vi "RT Driver VI.vi"(7 "Operation":T1, 11 "Device Reference in":T2 format="%.0x") -> (0 "Error Code":i32)   [LabVIEW 2021, in "FPGA Addon Engine.lvlib"]
uses:
  FPGA Addon Engine.lvlib
  <vilib>/NI VeriStand/Custom Device API/Custom Device Item Ref.ctl
  <vilib>/NI VeriStand/Custom Device API/Hardware Interface Driver VI Operation.ctl
  <vilib>/NI/NIVS Inline Async API/_VS Inline Async API/VS Inline Async API/Types/Error Handling Settings.ctl
  <vilib>/NI/NIVS Inline Async API/_VS Inline Async API/VS Inline Async API/VS Inline Async API.lvclass/VS Inline Async API.ctl
  <vilib>/NI/NIVS Inline Async API/_Data Access Engine/Data Access Engine/Data Access Engine.lvclass/Data Access Engine.ctl
  <vilib>/NI/NIVS Inline Async API/_Data Access Engine/Access Type Classes/Write/Write.lvclass/Write.ctl
  <vilib>/NI/NIVS Inline Async API/_Data Access Engine/Access Type Classes/ReadWrite/ReadWrite.lvclass/ReadWrite.ctl
  <vilib>/NI/NIVS Inline Async API/_Data Access Engine/Access Type Classes/Read/Read.lvclass/Read.ctl
  Addon Shared/SubVIs/FPGA Settings.vi
  SubVIs/Initialize Scalar Datatypes and Refs.vi
  <vilib>/NI/NIVS Inline Async API/_Data Access Engine/Data Access Engine/Methods/Data.Engine.Read Data from HW.vi
  <vilib>/NI/NIVS Inline Async API/_VS Inline Async API/Error Handling Process/SubVIs/Error.GetError.vi
  <vilib>/NI/NIVS Inline Async API/_Data Access Engine/Data Access Engine/Methods/Data.Engine.Write Data to HW.vi
  <vilib>/NI/NIVS Inline Async API/_Data Access Engine/Access Type Classes/ReadWrite/ReadWrite.EngineData.vi
  <vilib>/NI/NIVS Inline Async API/_Data Access Engine/Access Type Classes/Write/Write.EngineData.vi
  <vilib>/NI/NIVS Inline Async API/_Data Access Engine/Access Type Classes/Read/Read.EngineData.vi
  <vilib>/NI VeriStand/Custom Device API/NI VeriStand - Get Channel Value by Data Reference.vi
  <vilib>/NI VeriStand/Custom Device API/NI VeriStand - Set Channel Value by Data Reference.vi
  <vilib>/NI VeriStand/Custom Device API/NI VeriStand - Get Target Type.vi
  <vilib>/Utility/config.llb/Open Config Data.vi
  <vilib>/Utility/config.llb/Get Key Names.vi
  <vilib>/Utility/config.llb/Write Key.vi
  <vilib>/Utility/config.llb/Write Key (I32).vi
  <vilib>/Utility/config.llb/Close Config Data.vi
  <vilib>/NI VeriStand/Custom Device API/NI VeriStand - Get Item Property.vi
  <vilib>/NI VeriStand/Custom Device API/Get Item Property (Variant).vi
  <vilib>/NI VeriStand/Custom Device API/Get Item Property (Dependent File).vi
  <vilib>/NI VeriStand/Custom Device API/Get Item Property (Path).vi
  <vilib>/NI VeriStand/Custom Device API/Get Item Property (String).vi
  <vilib>/NI VeriStand/Custom Device API/Get Item Property (Boolean).vi
  <vilib>/NI VeriStand/Custom Device API/NI VeriStand - Set Item Property.vi
  <vilib>/NI VeriStand/Custom Device API/Set Item Property (Path).vi
  <vilib>/NI VeriStand/Custom Device API/Set Item Property (String).vi
  <vilib>/NI VeriStand/Custom Device API/Set Item Property (Boolean).vi
  APIs/FPGA Register IO/Utilities/Open FPGA Session.vi
  SubVIs/Initialize Input DMA Refs.vi
  SubVIs/Initialize Output DMA Refs.vi
  SubVIs/Initialize Scalar Datatype Classes.vi
  <vilib>/Utility/SystemLogging/Write to System Log.vi
  Processes/Input Registers Engine.vi
  Processes/Output Registers Engine.vi
  Processes/Output DMA Engine.vi
  Processes/Input DMA Engine.vi
  <vilib>/Utility/error.llb/Error Cluster From Error Code.vi
  <vilib>/RVI Host/nirviSupport.llb/nirviErrorClusterFromErrorCode.vi
  <vilib>/rvi/errors/niLvFpgaAdjustHostInterfaceError.vi
  <vilib>/NI VeriStand/Custom Device API/Global Data Refs.vi
  <vilib>/FPGAPlugInAG/Dynamic/niLvFpga_Close_Dynamic.vi
  <vilib>/NI VeriStand/Custom Device Waveform API/Multiple Waveforms Write (DBL)/Multiple Waveforms Write (DBL).lvclass
  <vilib>/NI VeriStand/Custom Device Waveform API/Single Waveform Read (DBL)/Single Waveform Read (DBL).lvclass
  <vilib>/NI/NIVS Inline Async API/_VS Inline Async API/VS Inline Async API/VS Inline Async API.lvclass
  <vilib>/rvi/interface/nirviMethod/nirviMethod.xnode
  <vilib>/rvi/interface/nirviCloseFPGA/nirviCloseFPGA.xnode
  <vilib>/NI VeriStand/Custom Device API/Custom Device API.lvlib
  <vilib>/rvi/interface/nirviMethod/StockFPGA_InlinedMethodWaitForSingleIRQ.vi
  <vilib>/FPGAPlugInAG/Dynamic/niLvFpga_WaitOnIrq_Dynamic.vi
  <vilib>/FPGAPlugInAG/Dynamic/niLvFpga_AcknowledgeIrq_Dynamic.vi
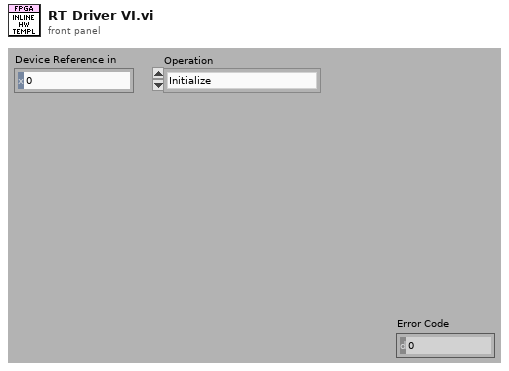
[diagram p1: front panel]
types:
  T1 = typedef "Custom Device API.lvlib/Hardware Interface Driver VI Operation.ctl" = enum16{"Initialize", "Start", "Read Data from HW", "Write Data to HW", "Close"}
  T2 = typedef "Custom Device API.lvlib/Custom Device Item Ref.ctl" = u64
  T3 = typedef "FPGA Addon Engine.lvlib/State Variables.ctl" = cluster{"FPGA Ref":refnum<k20>, "IncomingRegisters.Refs":T4[], "IncomingDMA.Refs":T7[], "OutgoingRegisters.Refs":T4[], "OutgoingDMA.Refs":T12[], "Compiled":T14}
  T4 = typedef "FPGA Addon Engine.lvlib/Register Settings.ctl" = cluster{"Name":string, "Data Type":T5, "session":u32, "Scalar Type":T6, "Index":i32, "Length":i32, "attributes":variant, "default value":variant}
  T5 = typedef "FPGA Addon Shared.lvlib/FPGA Addon Data Type.ctl" = enum8{"<Null>", "I8", "I16", "I32", "I64", "U8", "U16", "U32", "U64", "SGL", "Boolean", "Analog PWM In Settings", "Analog PWM In", "Digital PWM In Settings", "Digital PWM In", "Digital PWM Out", "Sine Out", "FXP", "FXP+/-24.5", "FXP+/-16.5", "FXP+/-32.8", "FXP+/-64.32", "FXP+/-16.7", "FXP+/-20.5", "FXP+/-27.5", "FXP+/-32.16", "FXP+16.3", "FXP+18.3", "Digital Static In", "Digital Static Out", "Digital Static In Settings", "Digital WSS Out", "Quad Encoder Settings", "Quad Encoder In", "Group"}
  T6 = typedef "FPGA Addon Shared.lvlib/Scalar Type.ctl" = enum16{"Standard", "Bitpacked"}
  T7 = typedef "FPGA Addon Engine.lvlib/DMA Input References.ctl" = cluster{"Addon Name":string, "Waveform Ref":refnum<class "Multiple Waveforms Write (DBL).lvclass">, "DMA Name":string, "DMA Settings":T8, "Refs":T11}
  T8 = typedef "FPGA Addon Shared.lvlib/DMA Settings.ctl" = cluster{"Number of Channels":u8, "Delacing Scheme":T9, "Update Rate":u32, "dt":dbl, "Mode":T10, "Number of Samples":u32, "DMA Host Buffer":u32}
  T9 = typedef "FPGA Addon Shared.lvlib/Delacing Scheme.ctl" = enum8{"Interleaved", "Bitpacked"}
  T10 = typedef "FPGA Addon Shared.lvlib/DMA Acquisition Mode.ctl" = enum8{"Continuous", "Triggered Finite"}
  T11 = typedef "FPGA Addon Engine.lvlib/DMA Input Refs.ctl" = cluster{"Data Type":T5, "DMA_SGL":refnum<k20>, "DMA_U64":refnum<k20>, "DMA_I64":refnum<k20>, "DMA_FXP+/-32.8":refnum<k20>, "DMA_FXP+/-64.32":refnum<k20>, "DMA_U32":refnum<k20>, "DMA_U16":refnum<k20>, "DMA_U8":refnum<k20>, "DMA_I32":refnum<k20>, "DMA_I16":refnum<k20>, "DMA_I8":refnum<k20>, "DMA_FXP+/-32.16":refnum<k20>}
  T12 = typedef "FPGA Addon Engine.lvlib/DMA Output References.ctl" = cluster{"Addon Name":string, "Waveforms":refnum<class "Single Waveform Read (DBL).lvclass">[], "DMA Name":string, "Refs":T13}
  T13 = typedef "FPGA Addon Engine.lvlib/DMA Output Refs.ctl" = cluster{"Data Type":T5, "DMA_SGL":refnum<k20>, "DMA_U64":refnum<k20>, "DMA_I64":refnum<k20>, "DMA_FXP+/-32.8":refnum<k20>, "DMA_FXP+/-64.32":refnum<k20>, "DMA_U32":refnum<k20>, "DMA_U16":refnum<k20>, "DMA_U8":refnum<k20>, "DMA_I32":refnum<k20>, "DMA_I16":refnum<k20>, "DMA_I8":refnum<k20>, "DMA_FXP+/-32.16":refnum<k20>}
  T14 = typedef "FPGA Addon Shared.lvlib/Compiled.Settings.ctl" = cluster{"Name":string, "IncomingRegisters.Settings":T15[], "IncomingRegisters.Refs":cluster{"Refs":T17[], "Values":dbl[]}, "OutgoingRegisters.Settings":T15[], "OutgoingRegisters.Refs":cluster{"Refs":T17[], "Values":dbl[]}, "Incoming.Size":i32, "Outgoing.Size":i32, "IncomingDMA.Settings":T19[], "OutgoingDMA.Settings":T19[], "FPGA.Settings":T21, "Target.Type":T22}
  T15 = typedef "FPGA Addon Shared.lvlib/Compiled.RegisterSettings.ctl" = cluster{"Scalar Type":T6, "Index":i32, "Length":i32, "Register":T16}
  T16 = typedef "FPGA Addon Shared.lvlib/Register Information.ctl" = cluster{"Name":string, "Data Type":T5, "Default Value":variant, "Attributes":variant}
  T17 = typedef "Custom Device API.lvlib/Block Data Reference.ctl" = cluster{"Data Reference":T18, "Offset":u64, "Length":u64}
  T18 = typedef "Custom Device API.lvlib/Data Reference.ctl" = i32
  T19 = typedef "FPGA Addon Shared.lvlib/Compiled.DMASettings.ctl" = cluster{"Name":string, "Data Type":T5, "DMA.Settings":T8, "DMA.VSRefs":T20[]}
  T20 = typedef "Custom Device API.lvlib/Waveform Data Reference.ctl" = i32
  T21 = typedef "FPGA Addon Shared.lvlib/FPGA Settings.ctl" = cluster{"Bitfile path":path, "RIO Device Address":string, "Group":bool}
  T22 = typedef "Custom Device API.lvlib/Custom Device Target Type.ctl" = enum16{"PharLap", "VxWorks", "Windows", "Linux_32_ARM", "Linux_x64"}
  T23 = cluster{"Vars":T3, "Async Read Data from HW":bool, "Async Data Write to HW":bool, "Async":refnum<class "VS Inline Async API.lvclass">}
  T24 = typedef "VS Inline Async API.lvlib/VS Inline Async API.lvclass/Error Handling Settings.ctl" = cluster{"Write to SystemLog (F)":bool}
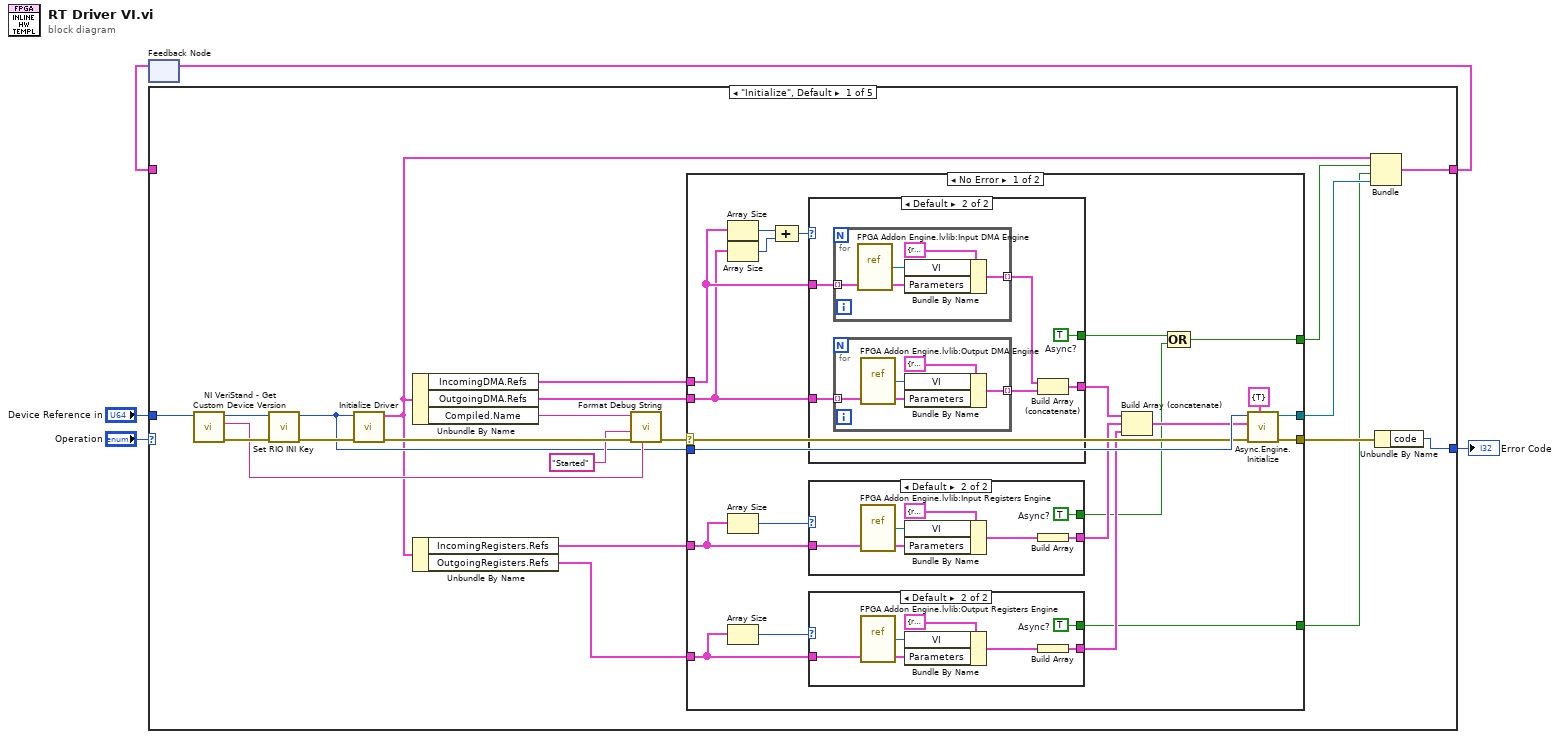
[diagram p0: block diagram]
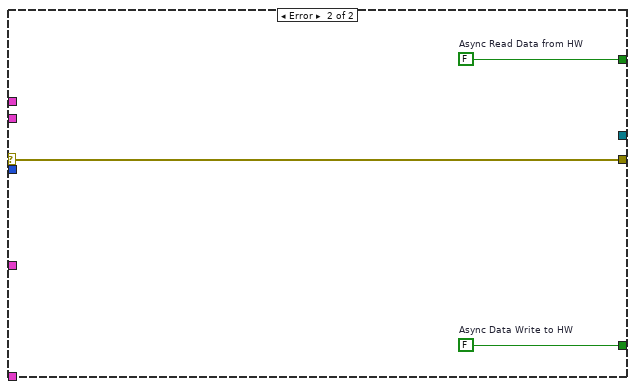
[diagram p5: hidden frame]
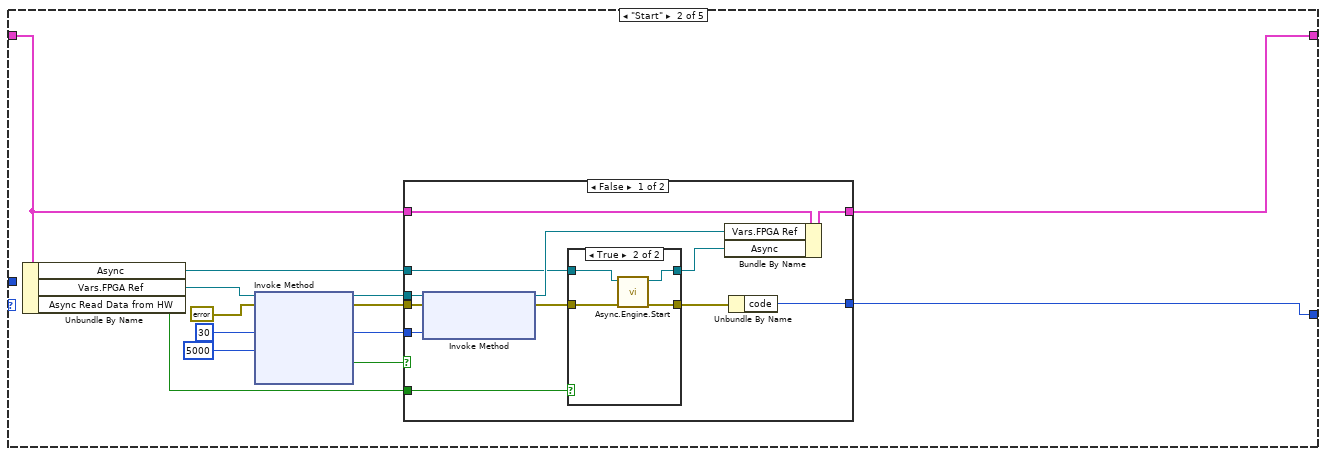
[diagram p6: hidden frame]
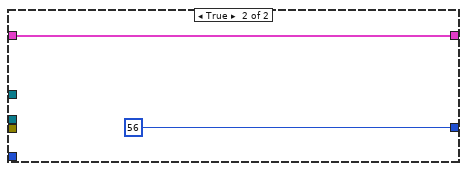
[diagram p8: hidden frame]
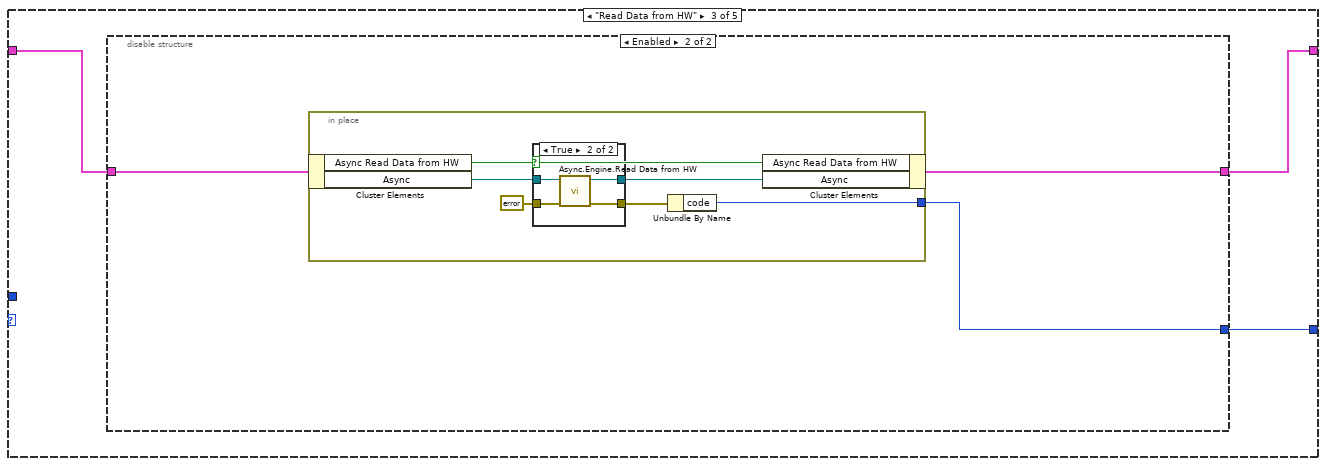
[diagram p9: hidden frame]
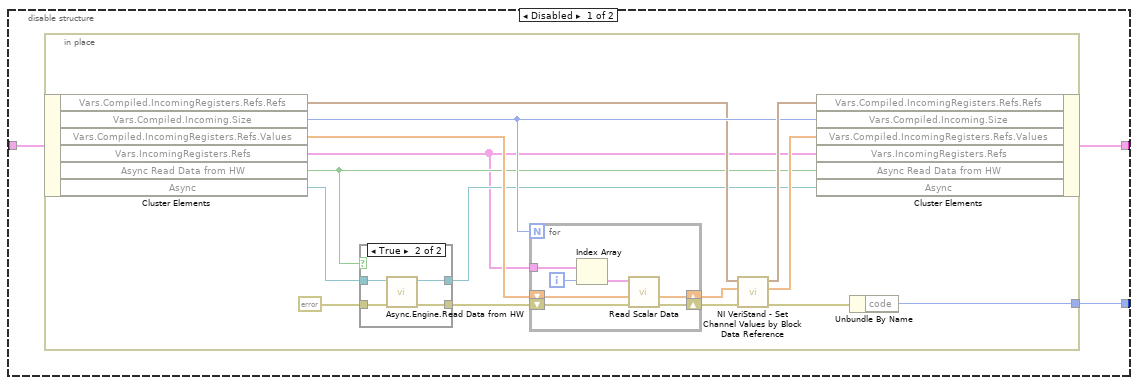
[diagram p10: hidden frame]
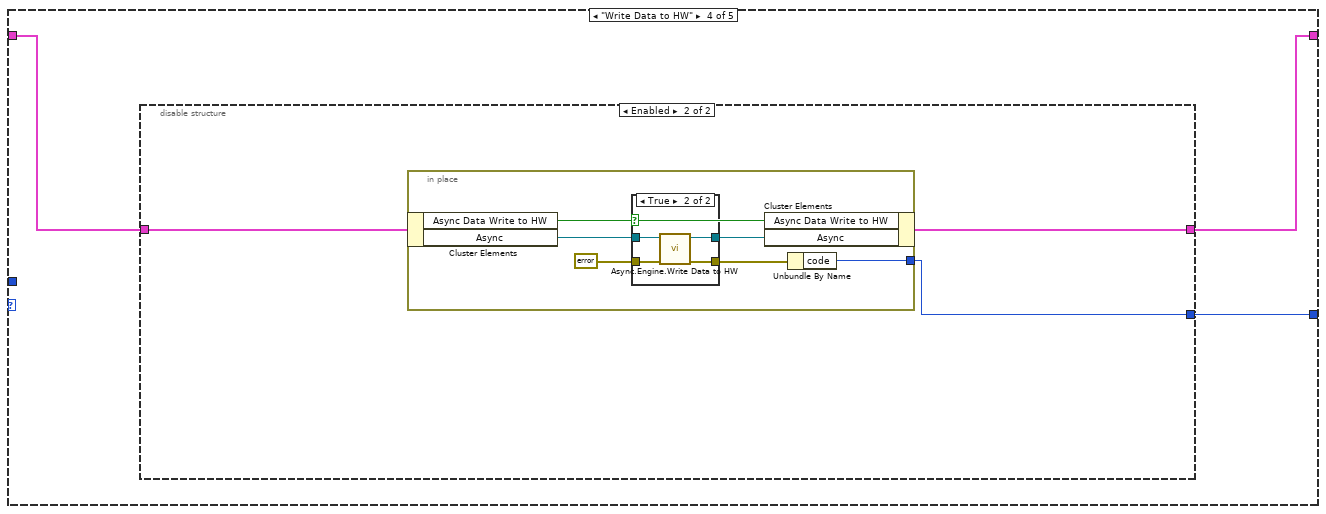
[diagram p13: hidden frame]
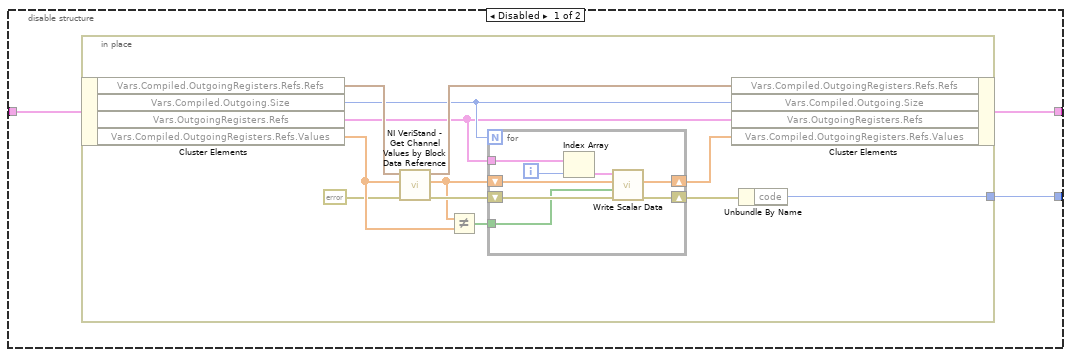
[diagram p14: hidden frame]
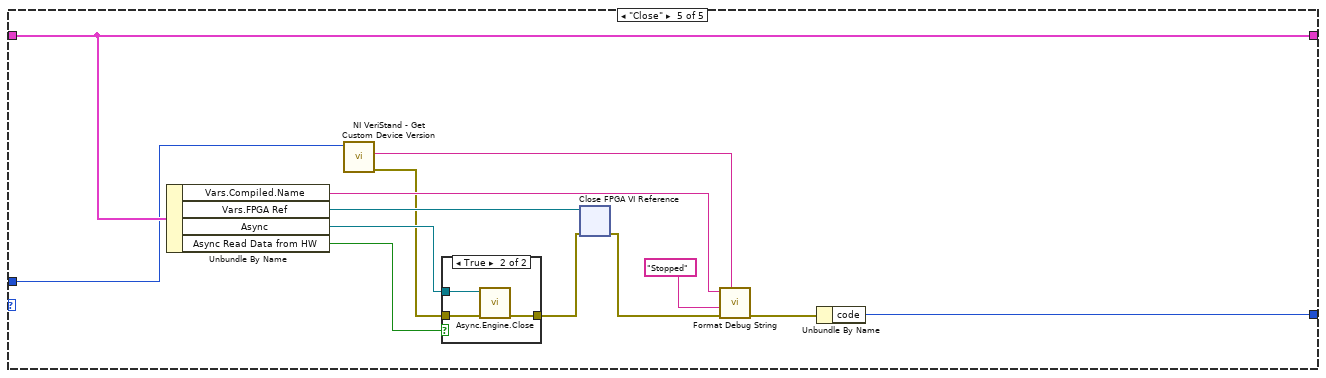
[diagram p16: hidden frame]
diagram:
  n1 = feedback #1() -> (w3:T23)  [unwired: 1 out]
  n2 = case shown="\"Initialize\", Default" "Operation" {
    tunnel: [w26 w87 w112 w160 w211] -> w4
    tunnel: w3 -> [_ w88 w110 w161 w211]
    tunnel: "Device Reference in" -> [w17 _ _ _ w206]
    tunnel: [w25 w89 w111 w159 w212] -> w1
    frame "Initialize", Default {
      n3 = call <vilib>:"NI VeriStand - Get Custom Device Version.vi"("Device Ref in"=w17) -> ("error out"=w18:errorcluster, "Value"=w15:string, "Device Ref out"=w11:T2)  [unwired: 8 in]
      n4 = call "Set RIO INI Key.vi"("error in (no error)"=w18, "Section Ref in"=w11) -> ("error out"=w24:errorcluster, "Section Ref out"=w10:T2)  [unwired: 8 in]
      n5 = call "Initialize Driver.vi"("error in (no error)"=w24, "Section Ref in"=w10) -> ("error out"=w16:errorcluster, "Vars"=w9:T3)  [unwired: 8 in]
      n6 = Unbundle By Name(w9) -> ("IncomingDMA.Refs"=w20:T7[], "OutgoingDMA.Refs"=w21:T12[], "Compiled.Name"=w14:string)
      n7 = Unbundle By Name(w9) -> ("IncomingRegisters.Refs"=w8:T4[], "OutgoingRegisters.Refs"=w7:T4[])
      n8 = call "Format Debug String.vi"("Version"=w15, "error in (no error)"=w16, "State"="Started" ("string"), "Name"=w14) -> ("error out"=w12:errorcluster)  [unwired: 7 in]
      n9 = case shown="No Error" w12 {
        selector: w12 -> [w45 w77]
        tunnel: [w48 w77] -> w23
        tunnel: [w47 _] -> w22
        tunnel: w21 -> [w42 _]
        tunnel: w20 -> [w43 _]
        tunnel: [w31 w76] -> w19
        tunnel: w10 -> [w46 _]
        tunnel: w7 -> [w38 _]
        tunnel: w8 -> [w39 _]
        tunnel: [w27 w75] -> w6
        frame No Error {
          n10 = Array Size(array=w43) -> (size(s)=w41:i32)
          n11 = Array Size(array=w42) -> (size(s)=w40:i32)
          n12 = Array Size(array=w39) -> (size(s)=w30:i32)
          n13 = Array Size(array=w38) -> (size(s)=w28:i32)
          n14 = Compound Arithmetic op=ADD(w41, w40) -> (w37:i32)
          n15 = case shown="Default" w37 {
            tunnel: w43 -> [_ w54]
            tunnel: w42 -> [_ w53]
            tunnel: [_ w50] -> w36
            tunnel: [_ w49] -> w32
            frame 0 {
            }
            frame Default {
              w49 = TRUE  # Async?
              n16 = for {
                tunnel: w54 -> [w61] mode=indexing
                tunnel: [w60] -> w51 mode=indexing
                n17 = vi-ref "FPGA Addon Engine.lvlib:Input DMA Engine.vi"() -> (w59:refnum<vi>)
                n18 = Bundle By Name(cluster=cluster{"VI":refnum<vi>, "Parameters":variant} {"VI"=refnum, "Parameters"=variant} ("Process"), "VI"=w59, "Parameters"=w61) -> (w60:cluster{"VI":refnum<vi>, "Parameters":variant})
              }
              n19 = for {
                tunnel: w53 -> [w55] mode=indexing
                tunnel: [w57] -> w52 mode=indexing
                n20 = vi-ref "FPGA Addon Engine.lvlib:Output DMA Engine.vi"() -> (w56:refnum<vi>)
                n21 = Bundle By Name(cluster=cluster{"VI":refnum<vi>, "Parameters":variant} {"VI"=refnum, "Parameters"=variant} ("Process"), "VI"=w56, "Parameters"=w55) -> (w57:cluster{"VI":refnum<vi>, "Parameters":variant})
              }
              n22 = Build Array (concatenate)(w51, w52) -> (w50:cluster{"VI":refnum<vi>, "Parameters":variant}[])
            }
          }
          n23 = case shown="Default" w30 {
            tunnel: w39 -> [_ w74]
            tunnel: [_ w70] -> w35
            tunnel: [_ w69] -> w29
            frame 0 {
            }
            frame Default {
              w69 = TRUE  # Async?
              n24 = vi-ref "FPGA Addon Engine.lvlib:Input Registers Engine.vi"() -> (w72:refnum<vi>)
              n25 = Bundle By Name(cluster=cluster{"VI":refnum<vi>, "Parameters":variant} {"VI"=refnum, "Parameters"=variant} ("Process"), "VI"=w72, "Parameters"=w74) -> (w71:cluster{"VI":refnum<vi>, "Parameters":variant})
              n26 = Build Array(w71) -> (w70:cluster{"VI":refnum<vi>, "Parameters":variant}[])
            }
          }
          n27 = case shown="Default" w28 {
            tunnel: w38 -> [_ w68]
            tunnel: [_ w64] -> w34
            tunnel: [_ w63] -> w27
            frame 0 {
            }
            frame Default {
              w63 = TRUE  # Async?
              n28 = vi-ref "FPGA Addon Engine.lvlib:Output Registers Engine.vi"() -> (w66:refnum<vi>)
              n29 = Bundle By Name(cluster=cluster{"VI":refnum<vi>, "Parameters":variant} {"VI"=refnum, "Parameters"=variant} ("Process"), "VI"=w66, "Parameters"=w68) -> (w65:cluster{"VI":refnum<vi>, "Parameters":variant})
              n30 = Build Array(w65) -> (w64:cluster{"VI":refnum<vi>, "Parameters":variant}[])
            }
          }
          n31 = Build Array (concatenate)(w36, w35, w34) -> (w33:cluster{"VI":refnum<vi>, "Parameters":variant}[])
          n32 = Compound Arithmetic op=OR(w32, w29) -> (w31:bool)
          n33 = call <vilib>:"Async.Engine.Initialize.vi"("Error Log Settings"=T24 {"Write to SystemLog (F)"=TRUE}, "error in (no error)"=w45, "Processes"=w33, "Custom Device Ref"=w46) -> ("error out"=w48:errorcluster, "Async"=w47:refnum<class "VS Inline Async API.lvclass">)  [unwired: 6 in]
        }
        frame Error {
          w75 = FALSE  # Async Data Write to HW
          w76 = FALSE  # Async Read Data from HW
        }
      }
      n34 = Bundle("Vars"=w9, "Async Read Data from HW"=w19, "Async Data Write to HW"=w6, "Async"=w22) -> (w26:T23)  [unwired: 1 out]
      n35 = Unbundle By Name(w23) -> ("code"=w25:i32)
    }
    frame "Start" {
      w83 = 30 ("IRQ Number(s)")
      n36 = Unbundle By Name(w88) -> ("Async"=w79:refnum<class "VS Inline Async API.lvclass">, "Vars.FPGA Ref"=w86:refnum<k20>, "Async Read Data from HW"=w81:bool)
      n37 = xnode "Invoke Method"("FPGA VI Reference In"=w86, "error in"=errorcluster {"status"=FALSE, "code"=0, "source"=""}, "IRQ Number(s)"=w83, "Timeout (ms)"=5000) -> ("FPGA VI Reference Out"=w85:refnum<k20>, "error out"=w84:errorcluster, "Timed Out"=w80:bool)  [unwired: 1 out]
      n38 = case shown="False" w80 {
        tunnel: [w101 56 ("code")] -> w89
        tunnel: w88 -> [w100 w109]
        tunnel: [w99 w109] -> w87
        tunnel: w85 -> [w98 _]
        tunnel: w84 -> [w97 _]
        tunnel: w83 -> [w96 _]
        tunnel: w81 -> [w93 _]
        tunnel: w79 -> [w92 _]
        frame False {
          n39 = xnode "Invoke Method"("FPGA VI Reference In"=w98, "error in"=w97, "IRQ Number(s)"=w96) -> ("FPGA VI Reference Out"=w95:refnum<k20>, "error out"=w90:errorcluster)
          n40 = case shown="True" w93 {
            tunnel: w90 -> [w103 w107]
            tunnel: [w103 w106] -> w94
            tunnel: w92 -> [w102 w105]
            tunnel: [w102 w104] -> w91
            frame False {
            }
            frame True {
              n41 = call <vilib>:"Async.Engine.Start.vi"("error in (no error)"=w107, "VS Inline Async API in"=w105) -> ("error out"=w106:errorcluster, "VS Inline Async API out"=w104:refnum<class "VS Inline Async API.lvclass">)  [unwired: 8 in]
            }
          }
          n42 = Bundle By Name(cluster=w100, "Vars.FPGA Ref"=w95, "Async"=w91) -> (w99:T23)
          n43 = Unbundle By Name(w94) -> ("code"=w101:i32)
        }
        frame True {
        }
      }
    }
    frame "Read Data from HW" {
      n44 = disable-structure shown="Enabled" {
        disable-tunnel: [w115 w145] -> w112
        disable-tunnel: [w114 w144] -> w111
        disable-tunnel: w110 -> [w113 w146]
        frame Disabled {
          n45 = in-place {
            in-place-border: [w122] -> w114
            n46 = in-place-cluster #2(w113) -> ("Vars.Compiled.IncomingRegisters.Refs.Refs"=w124:T17[], "Vars.Compiled.Incoming.Size"=w126:i32, "Vars.Compiled.IncomingRegisters.Refs.Values"=w130:dbl[], "Vars.IncomingRegisters.Refs"=w116:T4[], "Async Read Data from HW"=w118:bool, "Async"=w120:refnum<class "VS Inline Async API.lvclass">)
            n47 = case shown="True" w118 {
              tunnel: w120 -> [w132 w136]
              tunnel: [w131 w135] -> w121
              tunnel: [w132 w134] -> w119
              tunnel: errorcluster {"status"=FALSE, "code"=0, "source"=""} ("error in") -> [w131 w133]
              frame False {
              }
              frame True {
                n48 = call <vilib>:"Async.Engine.Read Data from HW.vi"("error in"=w133, "Async in"=w136) -> ("error out"=w135:errorcluster, "Async out"=w134:refnum<class "VS Inline Async API.lvclass">)  [unwired: 8 in]
              }
            }
            n49 = for {
              N: w126 -> [_]
              shift-right: [w137] -> w127
              shift-left: w130 -> [w138]
              shift-right: [w141] -> w125
              shift-left: w121 -> [w142]
              tunnel: w116 -> [w143]
              i -> [w139]
              n50 = Index Array(array=w143, index=w139) -> (element=w140:T4)
              n51 = call "Read Scalar Data.vi"("error in (no error)"=w142, "Values"=w138, "Cluster"=w140) -> ("error out"=w141:errorcluster, "Values"=w137:dbl[])  [unwired: 7 in]
            }
            n52 = call <vilib>:"NI VeriStand - Set Channel Values by Block Data Reference.vi"("error in (no error)"=w125, "Values Array in"=w127, "Block Data Ref"=w124) -> ("error out"=w123:errorcluster, "Values Array out"=w128:dbl[], "Block Data Ref dup"=w129:T17[])  [unwired: 6 in]
            n53 = in-place-cluster #2("Vars.Compiled.IncomingRegisters.Refs.Refs"=w129, "Vars.Compiled.Incoming.Size"=w126, "Vars.Compiled.IncomingRegisters.Refs.Values"=w128, "Vars.IncomingRegisters.Refs"=w116, "Async Read Data from HW"=w118, "Async"=w119) -> (w115:T23)
            n54 = Unbundle By Name(w123) -> ("code"=w122:i32)
          }
        }
        frame Enabled {
          n55 = in-place {
            in-place-border: [w152] -> w144
            n56 = in-place-cluster #3(w146) -> ("Async Read Data from HW"=w147:bool, "Async"=w151:refnum<class "VS Inline Async API.lvclass">)
            n57 = case shown="True" w147 {
              tunnel: w151 -> [w154 w158]
              tunnel: [w153 w157] -> w150
              tunnel: [w154 w156] -> w148
              tunnel: errorcluster {"status"=FALSE, "code"=0, "source"=""} ("error in") -> [w153 w155]
              frame False {
              }
              frame True {
                n58 = call <vilib>:"Async.Engine.Read Data from HW.vi"("error in"=w155, "Async in"=w158) -> ("error out"=w157:errorcluster, "Async out"=w156:refnum<class "VS Inline Async API.lvclass">)  [unwired: 8 in]
              }
            }
            n59 = Unbundle By Name(w150) -> ("code"=w152:i32)
            n60 = in-place-cluster #3("Async Read Data from HW"=w147, "Async"=w148) -> (w145:T23)
          }
        }
      }
    }
    frame "Write Data to HW" {
      n61 = disable-structure shown="Enabled" {
        disable-tunnel: w161 -> [w164 w187]
        disable-tunnel: [w163 w186] -> w160
        disable-tunnel: [w162 w185] -> w159
        frame Disabled {
          n62 = in-place {
            in-place-border: [w170] -> w162
            n63 = in-place-cluster #4(w164) -> ("Vars.Compiled.OutgoingRegisters.Refs.Refs"=w176:T17[], "Vars.Compiled.Outgoing.Size"=w172:i32, "Vars.OutgoingRegisters.Refs"=w165:T4[], "Vars.Compiled.OutgoingRegisters.Refs.Values"=w168:dbl[])
            n64 = call <vilib>:"NI VeriStand - Get Channel Values by Block Data Reference.vi"("error in (no error)"=errorcluster {"status"=FALSE, "code"=0, "source"=""} ("error in"), "Values Array in"=w168, "Block Data Ref"=w176) -> ("error out"=w173:errorcluster, "Values Array out"=w169:dbl[], "Block Data Ref dup"=w175:T17[])  [unwired: 6 in]
            n65 = Not Equal?(x=w169, y=w168) -> (x != y?=w167:bool[])
            n66 = for {
              N: w172 -> [_]
              shift-right: [w178] -> w174
              shift-left: w169 -> [w183]
              shift-right: [w179] -> w171
              shift-left: w173 -> [w184]
              tunnel: w167 -> [w177]
              tunnel: w165 -> [w182]
              i -> [w180]
              n67 = Index Array(array=w182, index=w180) -> (element=w181:T4)
              n68 = call "Write Scalar Data.vi"("error in (no error)"=w184, "Changed?"=w177, "Values"=w183, "Cluster"=w181) -> ("error out"=w179:errorcluster, "Values"=w178:dbl[])  [unwired: 6 in]
            }
            n69 = in-place-cluster #4("Vars.Compiled.OutgoingRegisters.Refs.Refs"=w175, "Vars.Compiled.Outgoing.Size"=w172, "Vars.OutgoingRegisters.Refs"=w165, "Vars.Compiled.OutgoingRegisters.Refs.Values"=w174) -> (w163:T23)
            n70 = Unbundle By Name(w171) -> ("code"=w170:i32)
          }
        }
        frame Enabled {
          n71 = in-place {
            in-place-border: [w193] -> w185
            n72 = in-place-cluster #5(w187) -> ("Async Data Write to HW"=w189:bool, "Async"=w191:refnum<class "VS Inline Async API.lvclass">)
            n73 = case shown="True" w189 {
              tunnel: [w194 w199] -> w192
              tunnel: w191 -> [w195 w198]
              tunnel: [w195 w197] -> w190
              tunnel: errorcluster {"status"=FALSE, "code"=0, "source"=""} ("error in (no error)") -> [w194 w196]
              frame False {
              }
              frame True {
                n74 = call <vilib>:"Async.Engine.Write Data to HW.vi"("error in (no error)"=w196, "VS Inline Async API in"=w198) -> ("error out"=w199:errorcluster, "VS Inline Async API out"=w197:refnum<class "VS Inline Async API.lvclass">)  [unwired: 8 in]
              }
            }
            n75 = in-place-cluster #5("Async Data Write to HW"=w189, "Async"=w190) -> (w186:T23)
            n76 = Unbundle By Name(w192) -> ("code"=w193:i32)
          }
        }
      }
    }
    frame "Close" {
      n77 = Unbundle By Name(w211) -> ("Vars.Compiled.Name"=w201:string, "Vars.FPGA Ref"=w209:refnum<k20>, "Async"=w207:refnum<class "VS Inline Async API.lvclass">, "Async Read Data from HW"=w208:bool)
      n78 = call <vilib>:"NI VeriStand - Get Custom Device Version.vi"("Device Ref in"=w206) -> ("error out"=w200:errorcluster, "Value"=w202:string)  [unwired: 8 in, 1 out]
      n79 = case shown="True" w208 {
        tunnel: [w213 w216] -> w210
        tunnel: w207 -> [_ w215]
        tunnel: w200 -> [w213 w214]
        frame False {
        }
        frame True {
          n80 = call <vilib>:"Async.Engine.Close.vi"("error in (no error)"=w214, "Async in"=w215) -> ("error out"=w216:errorcluster)  [unwired: 8 in, 1 out]
        }
      }
      n81 = xnode "Close FPGA VI Reference"("FPGA VI Reference In"=w209, "error in"=w210) -> ("error out"=w203:errorcluster)
      n82 = call "Format Debug String.vi"("Version"=w202, "error in (no error)"=w203, "State"="Stopped" ("string"), "Name"=w201) -> ("error out"=w204:errorcluster)  [unwired: 7 in]
      n83 = Unbundle By Name(w204) -> ("code"=w212:i32)
    }
  }
  "Error Code" <- w1
  n84 = feedback-in #1(w4) -> ()
